vi "TestExec.Configure Local Station ID Read and Dialog.vi"(9 "Dialog":bool, 10 "Station":T1={"Name"="UNDEFINED", "PN"="UNDEFINED", "SN"="UNDEFINED", "Location"="UNDEFINED"}, 11 "Config File":path) -> (1 "Changed":bool, 3 "Station Out":T1)   [LabVIEW 2018]
uses:
  Test Executive/Test Executive/Controls and Type Defs/TestExec.Station ID.ctl
  <vilib>/Utility/config.llb/Read Key (String).vi
  <vilib>/Utility/config.llb/Write Key (String).vi
  <vilib>/Utility/config.llb/NI_LVConfig.lvlib
panel:
  out "Tab Control":enum32{"Inputs", "Data", "Outputs"}(tab)=enum."Data"
  in  "Station  Config File":path
  in  "Changed":bool
  in  "Cancel":bool
  # "Local Station ID"
  # "Remote Configuration"
  # "(Optional)"
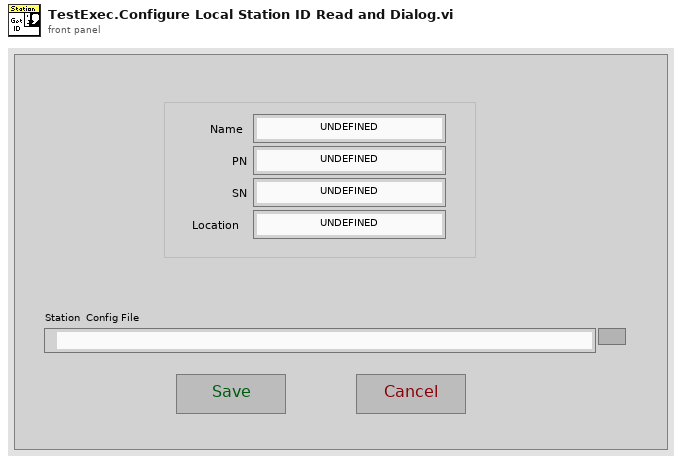
[diagram p1: front panel]
types:
  T1 = typedef "TestExec.Station ID.ctl" = cluster{"Name":string, "PN":string, "SN":string, "Location":string}
  T2 = enum32{"Invalid", "Standard", "Closed", "Hidden", "Minimized", "Maximized"}
  T3 = typedef "NI_LVConfig.lvlib/Config Data RefNum.ctl" = refnum<k1>
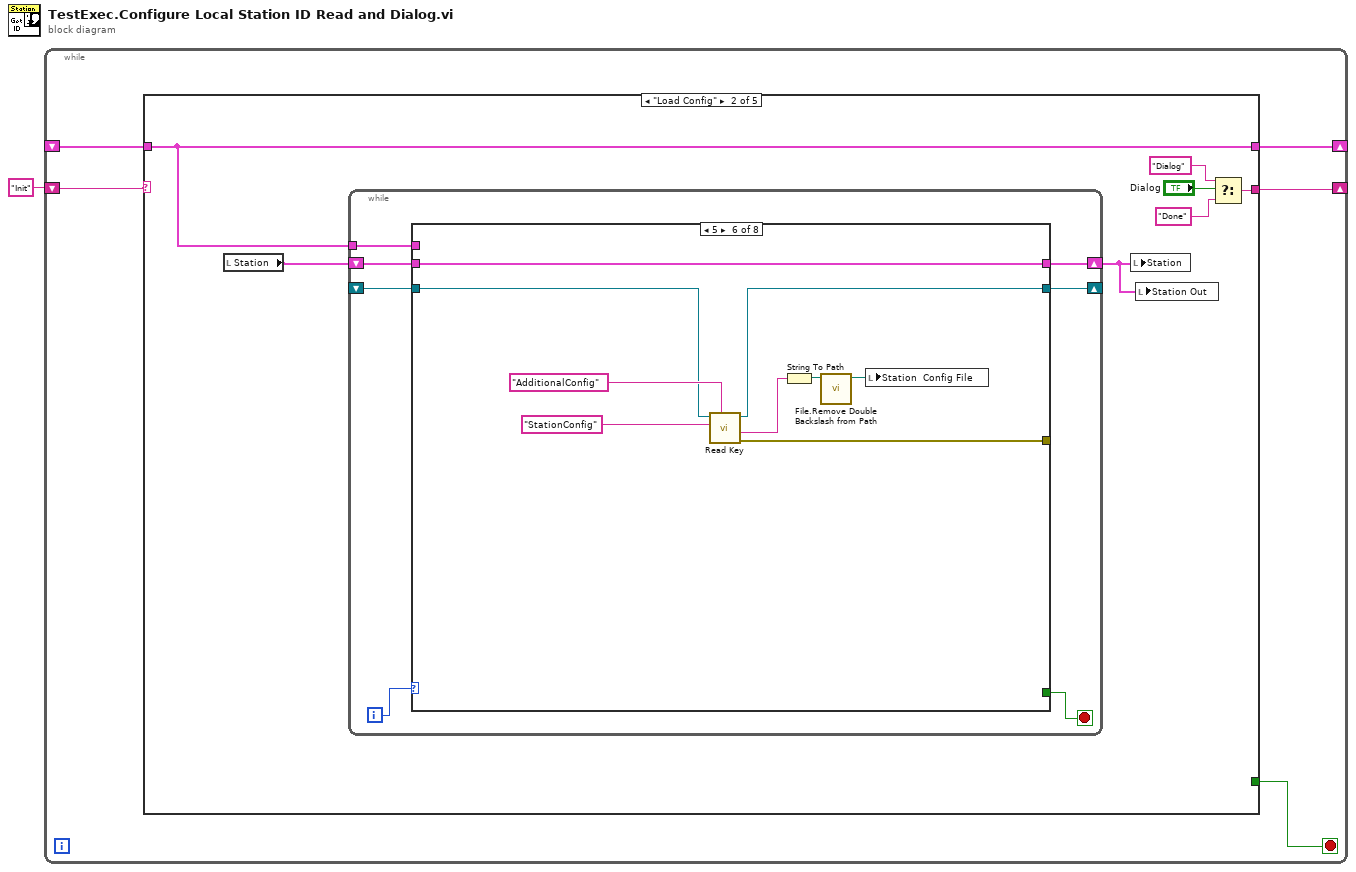
[diagram p0: block diagram]
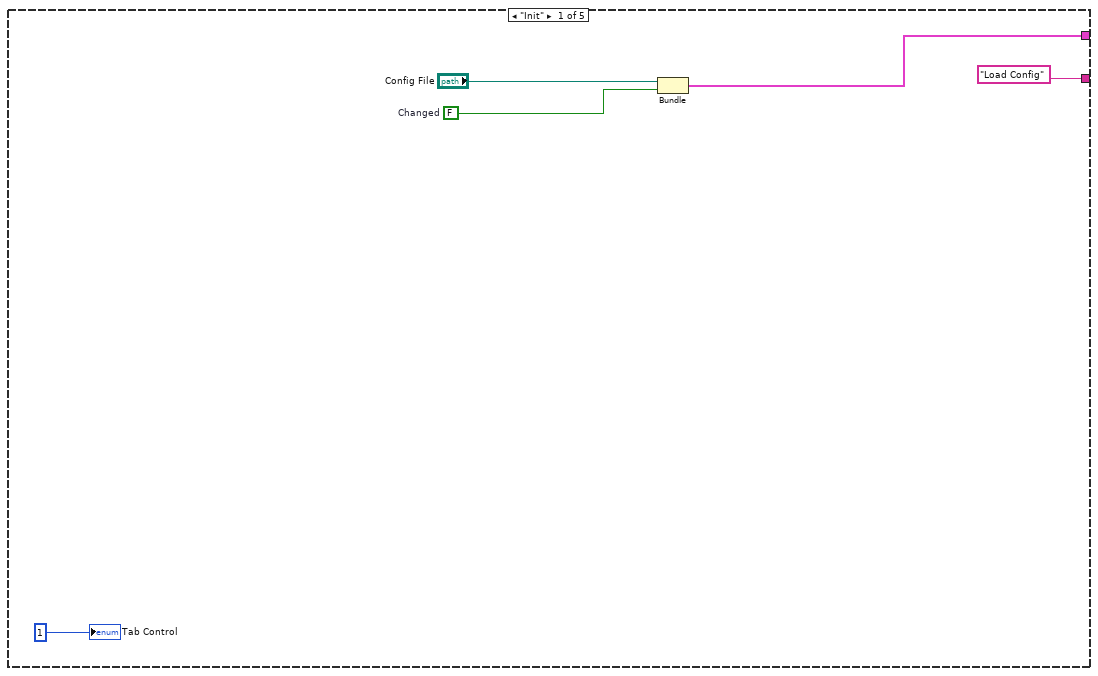
[diagram p2: hidden frame]
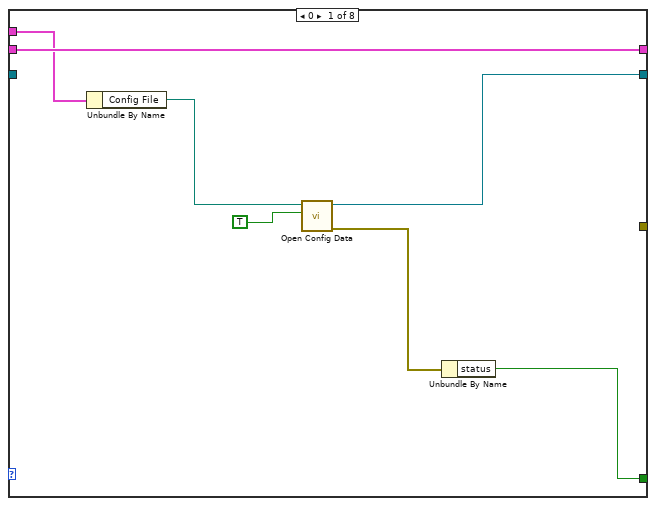
[diagram p3: hidden frame]
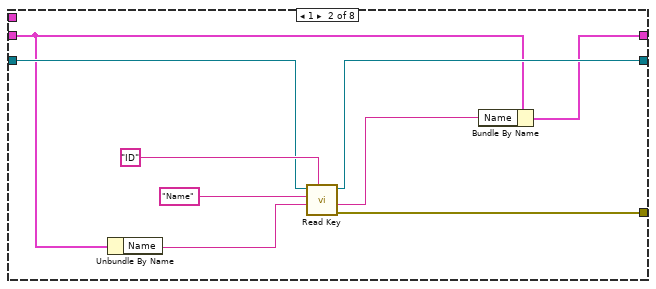
[diagram p4: hidden frame]
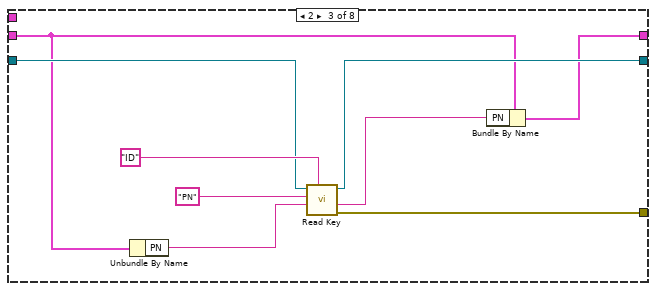
[diagram p5: hidden frame]
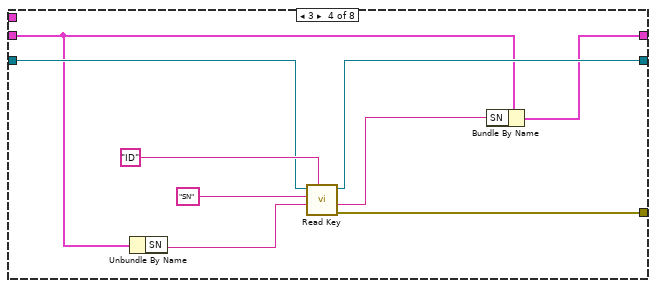
[diagram p6: hidden frame]
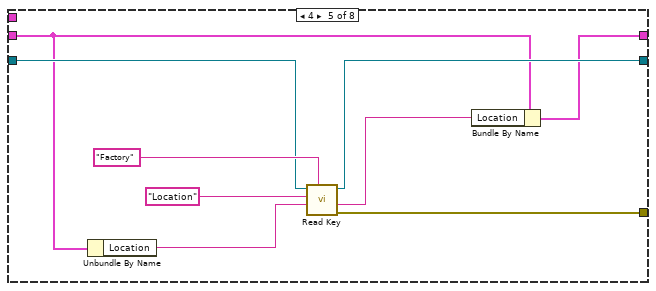
[diagram p7: hidden frame]
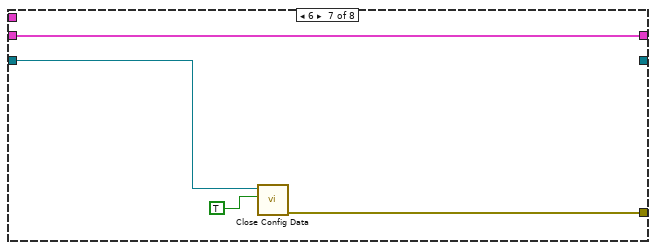
[diagram p8: hidden frame]
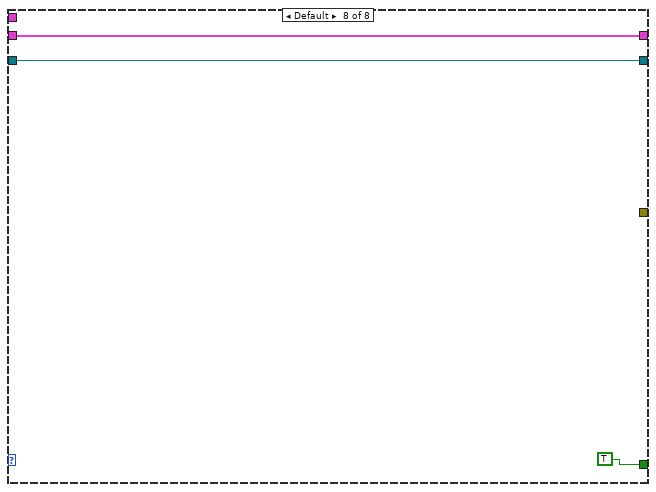
[diagram p9: hidden frame]
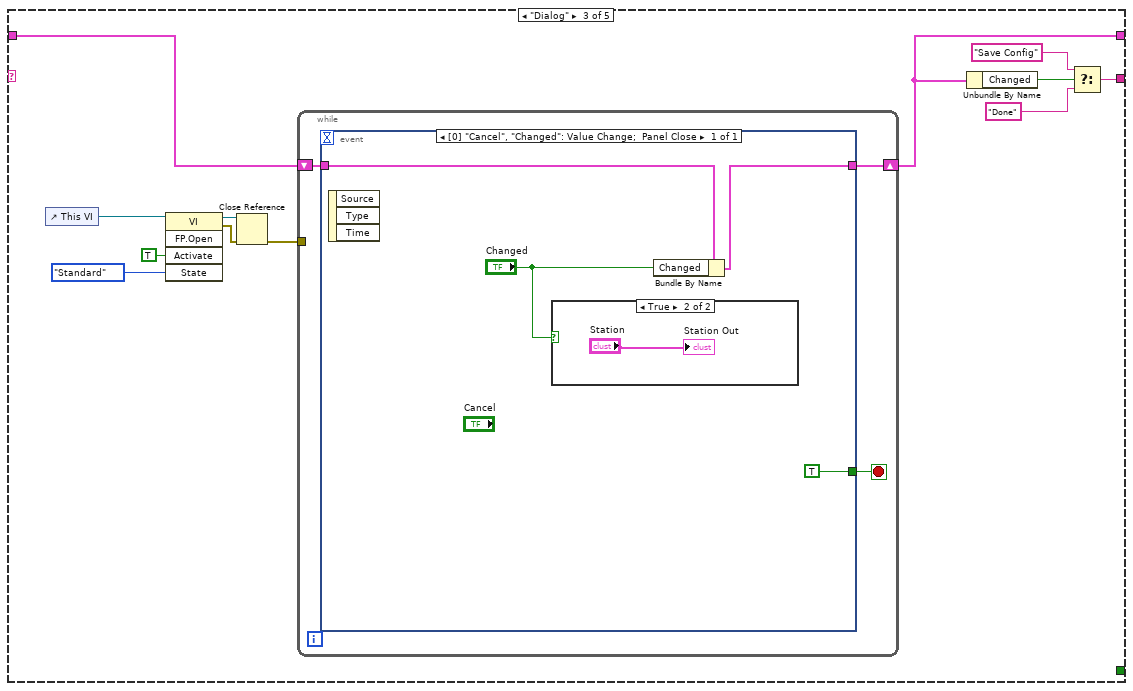
[diagram p10: hidden frame]
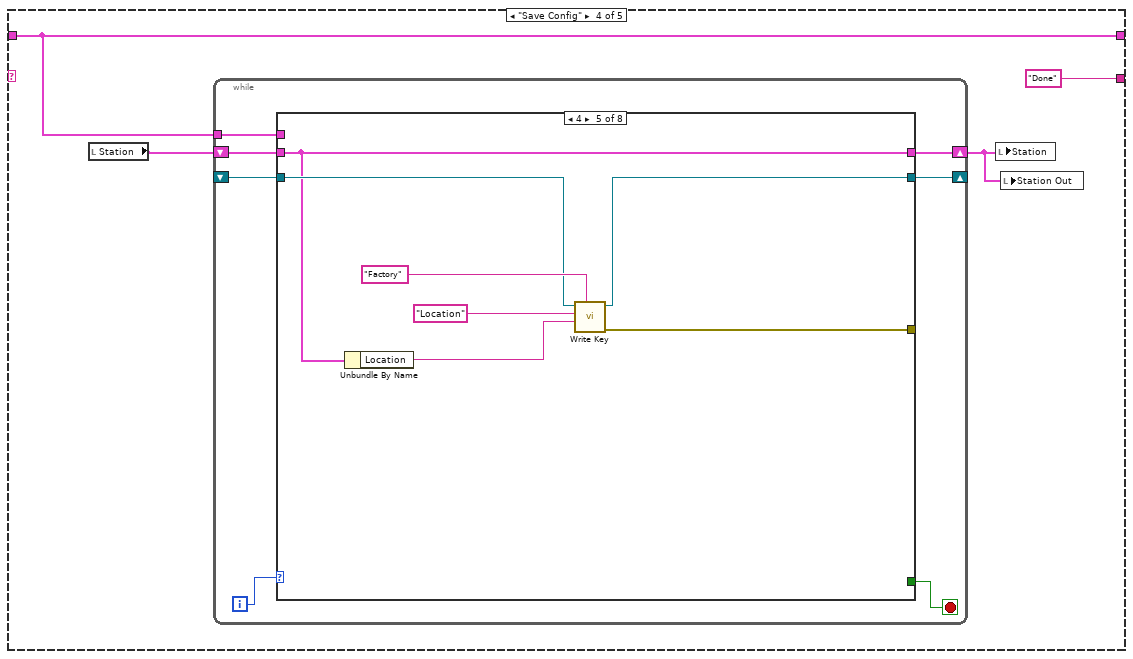
[diagram p12: hidden frame]
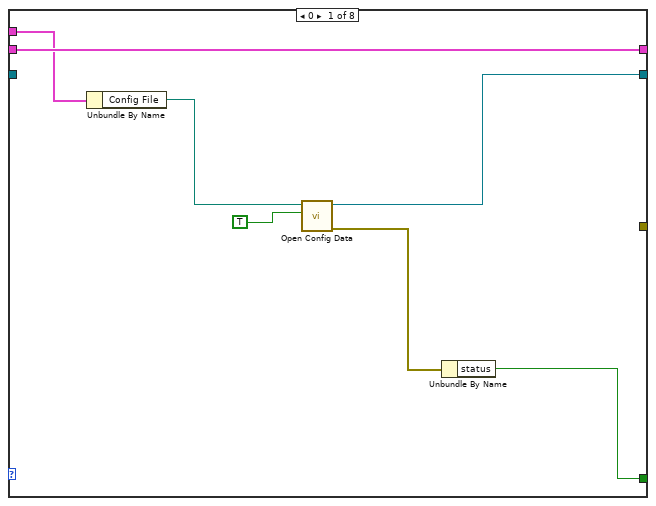
[diagram p13: hidden frame]
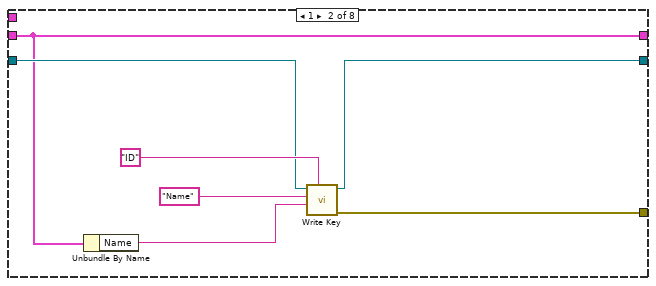
[diagram p14: hidden frame]
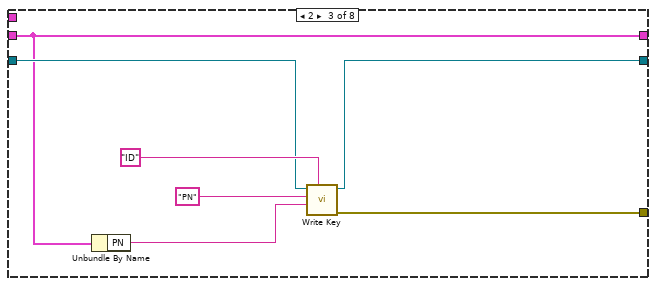
[diagram p15: hidden frame]
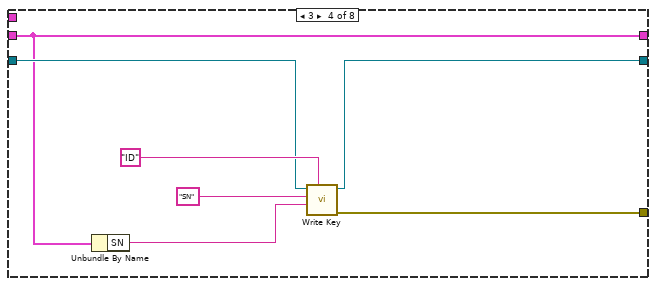
[diagram p16: hidden frame]
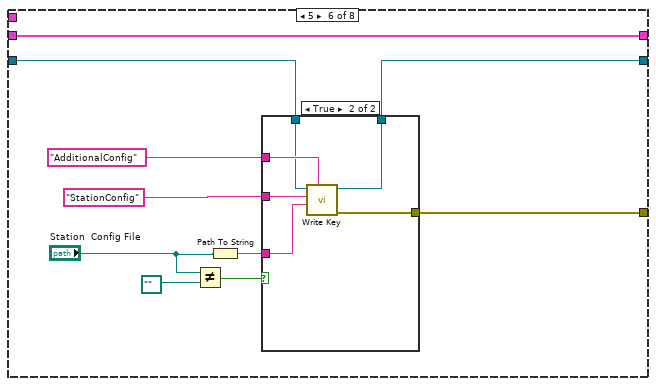
[diagram p17: hidden frame]
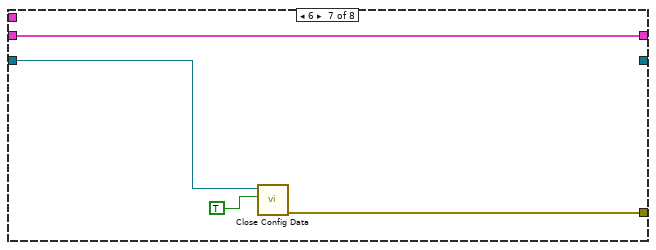
[diagram p19: hidden frame]
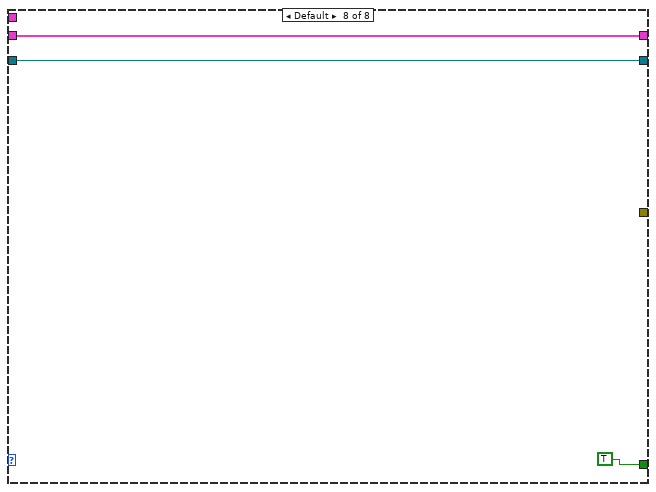
[diagram p20: hidden frame]
diagram:
  n1 = while {
    shift-right: [w4] -> _
    shift-left: _ -> [w6]
    shift-right: [w3] -> _
    shift-left: "Init" -> [w5]
    stop <- w2 stop-if-true
    n2 = case shown="\"Load Config\"" w5 {
      tunnel: w6 -> [_ w17 w90 w107 w179]
      tunnel: [w7 w17 w89 w107 w179] -> w4
      tunnel: ["Load Config" w15 w85 "Done" "Done"] -> w3
      tunnel: [_ _ _ _ TRUE] -> w2
      frame "Init" {
        w8 = FALSE  # Changed
        n3 = Bundle("Config File"="Config File", "Changed"=w8) -> (w7:cluster{"Config File":path, "Changed":bool})  [unwired: 1 in]
        "Tab Control" <- 1
      }
      frame "Load Config" {
        n4 = local read "Station"() -> (w18:T1)
        n5 = while {
          shift-right: [w22] -> _
          shift-left: _ -> [w23]
          shift-right: [w21] -> w12
          shift-left: w18 -> [w20]
          tunnel: w17 -> [w19]
          i -> [w25]
          stop <- w24 stop-if-true
          n6 = case shown="5" w25 {
            tunnel: [w30 _ _ _ _ _ _ TRUE] -> w24
            tunnel: w23 -> [_ w38 w47 w56 w65 w74 w81 w84]
            tunnel: [w32 w37 w46 w55 w64 w73 _ w84] -> w22
            tunnel: [_ w41 w50 w59 w68 w77 w80 _] -> _
            tunnel: [w28 w36 w45 w54 w63 w72 w78 w83] -> w21
            tunnel: w20 -> [w28 w34 w43 w52 w61 w72 w78 w83]
            tunnel: w19 -> [w27 _ _ _ _ _ _ _]
            frame 0 {
              n7 = Unbundle By Name(w27) -> ("Config File"=w26:path)
              n8 = call <vilib>:"Open Config Data.vi"("create file if necessary (T)"=TRUE, "configuration file path"=w26) -> ("error out"=w31:errorcluster, "refnum"=w32:T3)  [unwired: 7 in, 1 out]
              n9 = Unbundle By Name(w31) -> ("status"=w30:bool)
            }
            frame 1 {
              n10 = Unbundle By Name(w34) -> ("Name"=w33:string)
              n11 = call-poly <vilib>:"Read Key.vi"("section"="ID", "default value"=w33, "key"="Name" ("section"), "refnum"=w38) -> ("error out"=w41:errorcluster, "value"=w35:string, "refnum out"=w37:T3)  [unwired: 4 in, 1 out]
              n12 = Bundle By Name(cluster=w34, "Name"=w35) -> (w36:T1)
            }
            frame 2 {
              n13 = Unbundle By Name(w43) -> ("PN"=w42:string)
              n14 = call-poly <vilib>:"Read Key.vi"("section"="ID", "default value"=w42, "key"="PN" ("section"), "refnum"=w47) -> ("error out"=w50:errorcluster, "value"=w44:string, "refnum out"=w46:T3)  [unwired: 4 in, 1 out]
              n15 = Bundle By Name(cluster=w43, "PN"=w44) -> (w45:T1)
            }
            frame 3 {
              n16 = Unbundle By Name(w52) -> ("SN"=w51:string)
              n17 = call-poly <vilib>:"Read Key.vi"("section"="ID", "default value"=w51, "key"="SN" ("section"), "refnum"=w56) -> ("error out"=w59:errorcluster, "value"=w53:string, "refnum out"=w55:T3)  [unwired: 4 in, 1 out]
              n18 = Bundle By Name(cluster=w52, "SN"=w53) -> (w54:T1)
            }
            frame 4 {
              n19 = Unbundle By Name(w61) -> ("Location"=w60:string)
              n20 = call-poly <vilib>:"Read Key.vi"("section"="Factory", "default value"=w60, "key"="Location" ("section"), "refnum"=w65) -> ("error out"=w68:errorcluster, "value"=w62:string, "refnum out"=w64:T3)  [unwired: 4 in, 1 out]
              n21 = Bundle By Name(cluster=w61, "Location"=w62) -> (w63:T1)
            }
            frame 5 {
              n22 = call-poly <vilib>:"Read Key.vi"("section"="AdditionalConfig", "key"="StationConfig" ("section"), "refnum"=w74) -> ("error out"=w77:errorcluster, "value"=w71:string, "refnum out"=w73:T3)  [unwired: 5 in, 1 out]
              n23 = String To Path(string=w71) -> (path=w70:path)
              n24 = call "File.Remove Double Backslash from Path.vi"("Path"=w70) -> ("Path Out"=w69:path)  [unwired: 10 in]
              n25 = local write "Station  Config File"(w69) -> ()
            }
            frame 6 {
              n26 = call <vilib>:"Close Config Data.vi"("write file if changed (T)"=TRUE, "refnum"=w81) -> ("error out"=w80:errorcluster)  [unwired: 8 in, 1 out]
            }
            frame Default {
            }
          }
        }
        n27 = local write "Station"(w12) -> ()
        n28 = local write "Station Out"(w12) -> ()
        n29 = Select(t="Dialog", s="Dialog", f="Done") -> (s? t:f=w15:string)
      }
      frame "Dialog" {
        n30 = control-ref of="This VI"() -> (w96:refnum<vi>)
        n31 = invoke class="VI" method="FP.Open"(reference=w96, "Activate"=TRUE ("Activate?"), "State"=T2."Standard") -> (reference out=w93:refnum<vi>, error out=w92:errorcluster)  [unwired: 2 in, 3 out]
        n32 = Close Reference(reference=w93, error in (no error)=w92) -> (error out=w91:errorcluster)
        n33 = while {
          tunnel: w91 -> [_]
          shift-right: [w97] -> w89
          shift-left: w90 -> [w98]
          stop <- w99 stop-if-true
          n34 = event shown="[0] \"Cancel\", \"Changed\": Value Change;  Panel Close" {
            selector: _ -> [_]
            dyn-events: _ -> [_]
            timeout: _ -> [_]
            tunnel: [TRUE] -> w99
            tunnel: w98 -> [w102]
            tunnel: [w101] -> w97
            event "Cancel", "Changed": Value Change; Panel Close {
              n35 = event-data() -> ()  [unwired: 1 in, 3 out]
              n36 = case shown="True" "Changed" {
                frame False {
                }
                frame True {
                  "Station Out" <- "Station"
                }
              }
              n37 = Bundle By Name(cluster=w102, "Changed"="Changed") -> (w101:cluster{"Config File":path, "Changed":bool})
            }
          }
        }
        n38 = Unbundle By Name(w89) -> ("Changed"=w88:bool)
        n39 = Select(t="Save Config", s=w88, f="Done") -> (s? t:f=w85:string)
      }
      frame "Save Config" {
        n40 = local read "Station"() -> (w108:T1)
        n41 = while {
          shift-right: [w112] -> _
          shift-left: _ -> [w113]
          shift-right: [w111] -> w106
          shift-left: w108 -> [w110]
          tunnel: w107 -> [w109]
          i -> [w115]
          stop <- w114 stop-if-true
          n42 = case shown="4" w115 {
            tunnel: [w120 _ _ _ _ _ _ TRUE] -> w114
            tunnel: w113 -> [_ w126 w133 w140 w147 w157 w171 w174]
            tunnel: [w122 w125 w132 w139 w146 w156 _ w174] -> w112
            tunnel: [_ w129 w136 w143 w150 w160 w170 _] -> _
            tunnel: [w118 w123 w130 w137 w144 w155 w168 w173] -> w111
            tunnel: w110 -> [w118 w123 w130 w137 w144 w155 w168 w173]
            tunnel: w109 -> [w117 _ _ _ _ _ _ _]
            frame 0 {
              n43 = Unbundle By Name(w117) -> ("Config File"=w116:path)
              n44 = call <vilib>:"Open Config Data.vi"("create file if necessary (T)"=TRUE, "configuration file path"=w116) -> ("error out"=w121:errorcluster, "refnum"=w122:T3)  [unwired: 7 in, 1 out]
              n45 = Unbundle By Name(w121) -> ("status"=w120:bool)
            }
            frame 1 {
              n46 = Unbundle By Name(w123) -> ("Name"=w124:string)
              n47 = call-poly <vilib>:"Write Key.vi"("section"="ID", "value"=w124, "key"="Name" ("section"), "refnum"=w126) -> ("error out"=w129:errorcluster, "refnum out"=w125:T3)  [unwired: 5 in, 1 out]
            }
            frame 2 {
              n48 = Unbundle By Name(w130) -> ("PN"=w131:string)
              n49 = call-poly <vilib>:"Write Key.vi"("section"="ID", "value"=w131, "key"="PN" ("section"), "refnum"=w133) -> ("error out"=w136:errorcluster, "refnum out"=w132:T3)  [unwired: 5 in, 1 out]
            }
            frame 3 {
              n50 = Unbundle By Name(w137) -> ("SN"=w138:string)
              n51 = call-poly <vilib>:"Write Key.vi"("section"="ID", "value"=w138, "key"="SN" ("section"), "refnum"=w140) -> ("error out"=w143:errorcluster, "refnum out"=w139:T3)  [unwired: 5 in, 1 out]
            }
            frame 4 {
              n52 = Unbundle By Name(w144) -> ("Location"=w145:string)
              n53 = call-poly <vilib>:"Write Key.vi"("section"="Factory", "value"=w145, "key"="Location" ("section"), "refnum"=w147) -> ("error out"=w150:errorcluster, "refnum out"=w146:T3)  [unwired: 5 in, 1 out]
            }
            frame 5 {
              n54 = Not Equal?(x="Station  Config File", y=path "") -> (x != y?=w153:bool)
              n55 = Path To String(path="Station  Config File") -> (string=w151:string)
              n56 = case shown="True" w153 {
                tunnel: [_ w167] -> w160
                tunnel: "AdditionalConfig" ("section") -> [_ w166]
                tunnel: "StationConfig" ("section") -> [_ w165]
                tunnel: w157 -> [w161 w164]
                tunnel: [w161 w163] -> w156
                tunnel: w151 -> [_ w162]
                frame False {
                }
                frame True {
                  n57 = call-poly <vilib>:"Write Key.vi"("section"=w166, "value"=w162, "key"=w165, "refnum"=w164) -> ("error out"=w167:errorcluster, "refnum out"=w163:T3)  [unwired: 5 in, 1 out]
                }
              }
            }
            frame 6 {
              n58 = call <vilib>:"Close Config Data.vi"("write file if changed (T)"=TRUE, "refnum"=w171) -> ("error out"=w170:errorcluster)  [unwired: 8 in, 1 out]
            }
            frame Default {
            }
          }
        }
        n59 = local write "Station"(w106) -> ()
        n60 = local write "Station Out"(w106) -> ()
      }
      frame "Done", Default {
        w176 = TRUE  # Normal(T)/Debug(F)
        n61 = Unbundle By Name(w179) -> ("Changed"=→"Changed":bool)
        n62 = local read "Dialog"() -> (w177:bool)
        n63 = And(x=w177, y=w176) -> (x .and. y?=w175:bool)
        n64 = case shown="True" w175 {
          tunnel: [_ w182] -> _
          frame False {
          }
          frame True {
            n65 = control-ref of="This VI"() -> (w185:refnum<vi>)
            n66 = invoke class="VI" method="FP.Close"(reference=w185) -> (reference out=w184:refnum<vi>, error out=w183:errorcluster)  [unwired: 2 in, 1 out]
            n67 = Close Reference(reference=w184, error in (no error)=w183) -> (error out=w182:errorcluster)
          }
        }
      }
    }
  }
